vi "Rinocloud_HTTP_upload_file.vi"(4 "local storage":T1={"Store locally"=TRUE, "ancestor array"=[], "Store metadata"=TRUE}, 5 "Extra metadata array":T3(array[cluster])=[{"Attribute"="", "Value"="", "Data type"=enum."<null>"}, {"Attribute"="Amplitude", "Value"="10", "Data type"=enum."<null>"}], 6 "Path in":path, 7 "Parent ID":string, 8 "error in (no error)":errorcluster, 9 "Notes":string, 10 "Tags":string, 11 "Name":string) -> (0 "error out":errorcluster, 2 "Path out":path, 3 "Status":T2={"headers"="", "body"="", "ID"="", "Saved"=TRUE})   [LabVIEW 2011, in "Rinocloud Library.lvlib"]
uses:
  Rinocloud Library.lvlib
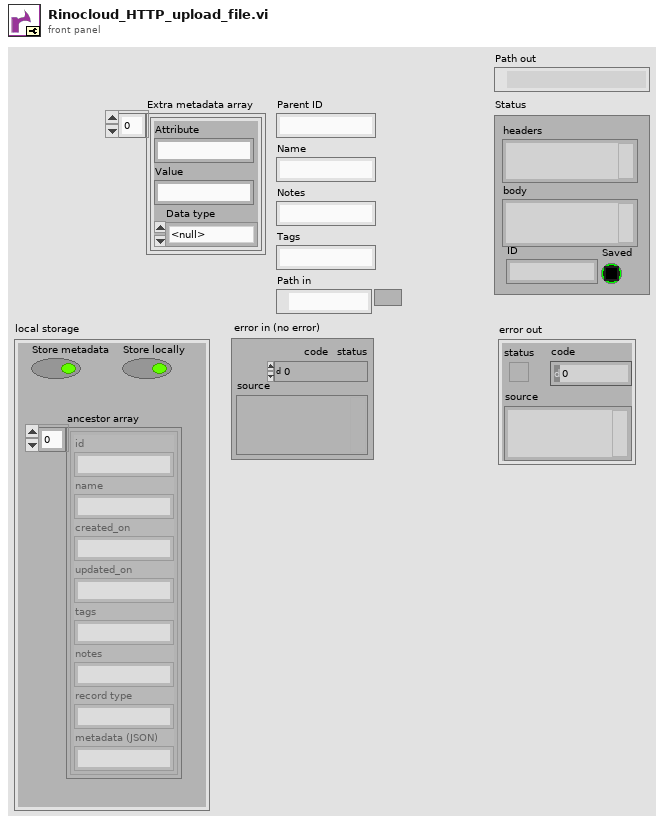
[diagram p1: front panel]
types:
  T1 = cluster{"Store locally":bool, "ancestor array":cluster{"id":string, "name":string, "created_on":string, "updated_on":string, "tags":string, "notes":string, "record type":string, "metadata (JSON)":string}[], "Store metadata":bool}
  T2 = cluster{"headers":string, "body":string, "ID":string, "Saved":bool}
  T3 = cluster{"Attribute":string, "Value":string, "Data type":enum16{"Numeric", "String", "1D array of strings", "1D array of doubles", "Data JSON string", "<null>"}}[]
  T4 = cluster{"Name":string, "Notes":string, "Tags":string}
  T5 = cluster{"id":string, "name":string, "created_on":string, "updated_on":string, "tags":string, "notes":string, "record type":string, "metadata (JSON)":string}[]
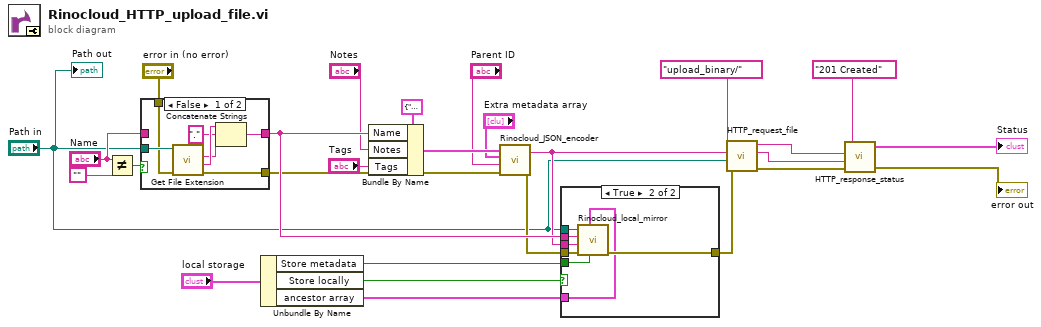
[diagram p0: block diagram]
diagram:
  n1 = Not Equal?(x="Name", y="") -> (x != y?=w17:bool)
  n2 = case shown="False" w17 {
    tunnel: [w33 w36] -> w22
    tunnel: "Name" -> [_ w36]
    tunnel: "Path in" -> [w34 _]
    tunnel: "error in (no error)" -> [w29 w35]
    tunnel: [w28 w35] -> w20
    frame False {
      n3 = call <vilib>:"Get File Extension.vi"("error in (no error)"=w29, "file"=w34) -> ("error out"=w28:errorcluster, "filename without extension"=w32:string, "lowercase file extension"=w30:string)  [unwired: 5 in, 2 out]
      n4 = Concatenate Strings(w32, "." ("string"), w30) -> (w33:string)
    }
    frame True {
    }
  }
  n5 = Unbundle By Name("local storage") -> ("Store metadata"=w1:bool, "Store locally"=w3:bool, "ancestor array"=w2:T5)
  n6 = Bundle By Name(cluster=T4 {"Name"="", "Notes"="", "Tags"=""} ("Metadata"), "Name"=w22, "Notes"="Notes", "Tags"="Tags") -> (w13:T4)
  n7 = call "Rinocloud_JSON_encoder.vi"("Metadata"=w13, "Extra metadata array"="Extra metadata array", "parent ID"="Parent ID", "error in (no error)"=w20) -> ("JSON payload"=w8:string, "error out"=w21:errorcluster)  [unwired: 1 in]
  n8 = case shown="True" w3 {
    tunnel: w22 -> [_ w44]
    tunnel: w21 -> [w37 w43]
    tunnel: [w37 w42] -> w9
    tunnel: w8 -> [_ w41]
    tunnel: "Path in" -> [_ w40]
    tunnel: w2 -> [_ w39]
    tunnel: w1 -> [_ w38]
    frame False {
    }
    frame True {
      n9 = call "Rinocloud_local_mirror.vi"("Store metadata"=w38, "ancestor array"=w39, "error in"=w43, "JSON payload"=w41, "file name"=w44, "file path"=w40) -> ("error out"=w42:errorcluster)  [unwired: 5 in]
    }
  }
  n10 = call "HTTP_request_file.vi"("error in (no error)"=w9, "Path"="Path in", "JSON payload"=w8, "Endpoint"="upload_binary/") -> ("error out"=w25:errorcluster, "Body"=w27:string, "Headers"=w26:string)  [unwired: 1 in]
  n11 = call "HTTP_response_status.vi"("error in (no error)"=w25, "body"=w27, "headers"=w26, "HTTP status"="201 Created") -> ("error out"=→"error out":errorcluster, "Status"=→"Status":T2)  [unwired: 1 in]
  "Path out" <- "Path in"
